vi "Init_Test.vi"(8 "error in (no error)":errorcluster caption="entrée d'erreur (pas d'erreur)", 11 "Flash_Jlink en entrée":refnum<class "Flash_Jlink.lvclass">) -> (0 "error out":errorcluster caption="sortie d'erreur", 3 "Flash_Jlink en sortie":refnum<class "Flash_Jlink.lvclass">)   [LabVIEW 2020, in "Library Test.lvlib" / "Flash_Jlink.lvclass"]
uses:
  Flash_Jlink.lvclass
  C:/Users/ngarcin/OneDrive - Altyor/Standard TB/Class/Test/Test (Default)/Test (Default).lvclass
  Commun VI/TypeDef/Commande Test/Commande Type Test.ctl
  Commun VI/TypeDef/Commande Test/Commande Value Type.ctl
  Flash_Jlink.lvclass/Flash_Jlink.ctl
  Test_Without_Instr/Test_Without_Inst.lvclass
  Process/Process (Default)/Process (Default).lvclass
  Commun VI/Library Commun.lvlib
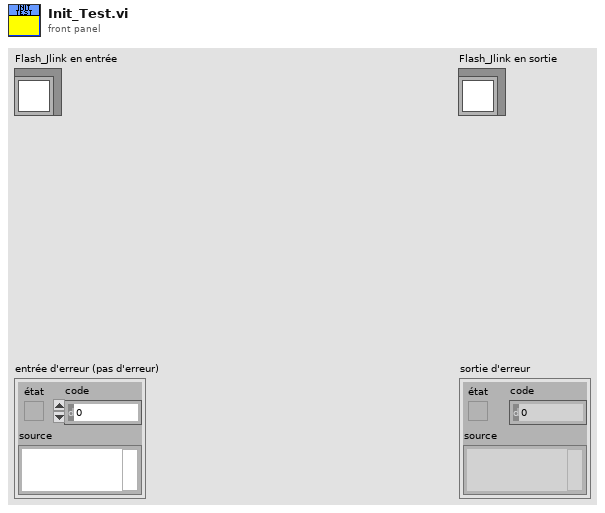
[diagram p1: front panel]
types:
  T1 = typedef "Library Commun.lvlib/Commande Value Type.ctl" = enum16{"None", "String", "Number", "Timestamp", "Boolean", "Array"}
  T2 = typedef "Library Commun.lvlib/Commande Type Test.ctl" = enum16{"Function", "Test", "Calculation"}
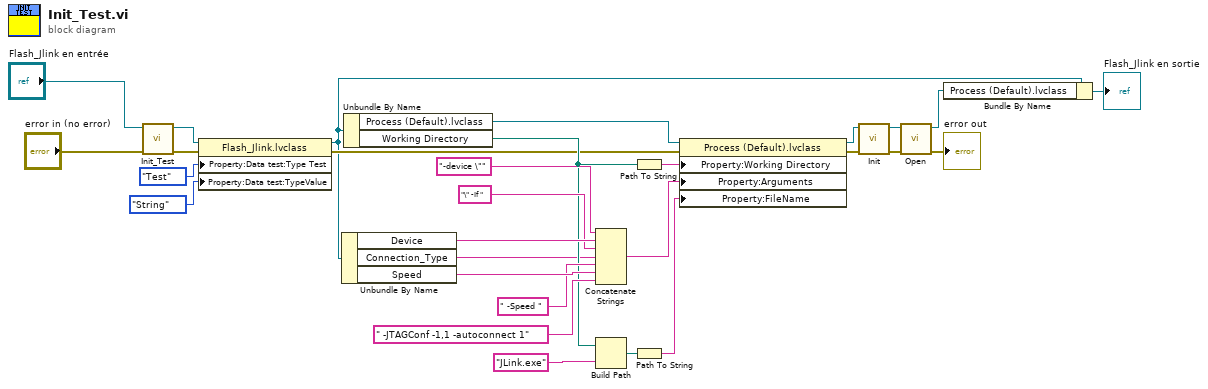
[diagram p0: block diagram]
diagram:
  n1 = call-parent "Init_Test.vi"("error in (no error)"="error in (no error)", "Test_Without_Inst en entrée"="Flash_Jlink en entrée") -> ("error out"=w4:errorcluster, "Test_Without_Inst en sortie"=w5:refnum<class "Flash_Jlink.lvclass">)  [unwired: 8 in]
  n2 = property class="Flash_Jlink.lvclass"(reference=w5, error in=w4, "Property:Data test:Type Test"=Commande_Type_Test."Test" ("Type Test"), "Property:Data test:TypeValue"=Commande_Value_Type."String" ("TypeValue")) -> (reference out=w2:refnum<class "Flash_Jlink.lvclass">, error out=w3:errorcluster)
  n3 = Unbundle By Name(w2) -> ("Device"=w18:string, "Connection_Type"=w1:string, "Speed"=w15:string)
  n4 = Unbundle By Name(w2) -> ("Process (Default).lvclass"=w27:refnum<class "Process (Default).lvclass">, "Working Directory"=w8:path)
  n5 = Concatenate Strings("-device \"" ("FileName"), w18, "\" -If " ("FileName"), w1, " -Speed " ("FileName"), w15, " -JTAGConf -1,1 -autoconnect 1" ("FileName")) -> (w12:string)
  n6 = Build Path(base path=w8, name or relative path="JLink.exe" ("nom ou chemin relatif")) -> (appended path=w19:path)
  n7 = Path To String(path=w8) -> (string=w11:string)
  n8 = Path To String(path=w19) -> (string=w9:string)
  n9 = property class="Process (Default).lvclass"(reference=w27, error in=w3, "Property:Working Directory"=w11, "Property:Arguments"=w12, "Property:FileName"=w9) -> (reference out=w26:refnum<class "Process (Default).lvclass">, error out=w10:errorcluster)
  n10 = call-dynamic "Init.vi"("error in (no error)"=w10, "Process (Default) en entrée"=w26) -> ("error out"=w24:errorcluster, "Process (Default) en sortie"=w22:refnum<class "Process (Default).lvclass">)  [unwired: 8 in]
  n11 = call-dynamic "Open.vi"("error in (no error)"=w24, "Process (Default) en entrée"=w22) -> ("error out"=→"error out":errorcluster, "Process (Default) en sortie"=w21:refnum<class "Process (Default).lvclass">)  [unwired: 8 in]
  n12 = Bundle By Name(cluster=w2, "Process (Default).lvclass"=w21) -> (→"Flash_Jlink en sortie":refnum<class "Flash_Jlink.lvclass">)
